vi "OE1022_Configure Input Filter.vi"(7 "OE1022_Configure Input Filter":T1 {"Input Notch Filter" items=["None"=0, "50Hz"=1, "100Hz"=3, "Both"=2]; "Input Coupling" items=["AC", "DC"]; "Input Shield Grounding" items=["Float", "Ground"]; "Input Source" items=["A", "A-B", "I-1M", "I-100M"]}, 8 "Error in (no error)":errorcluster caption="error out（no error）", 9 "Remote Mode":u16(ring) items=["USB"=0, "GPIB"=2], 11 "VISA resource name":refnum<visa-resource-name>) -> (0 "Error out":errorcluster caption="error out", 1 "Output String":string, 3 "VISA resource  out":refnum<visa-resource-name>)   [LabVIEW 2011]
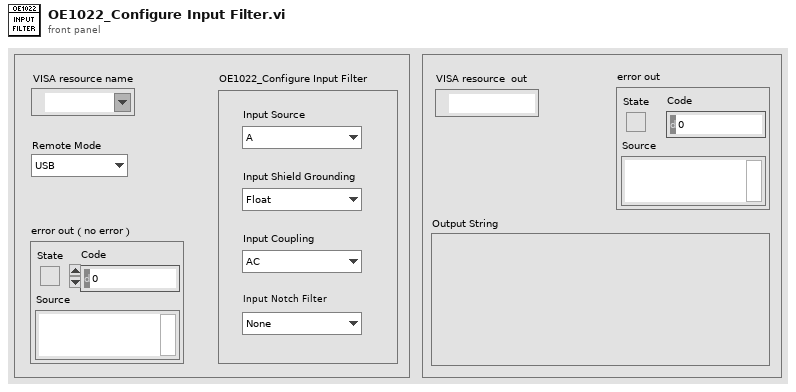
[diagram p1: front panel]
types:
  T1 = cluster{"Input Source":u16, "Input Shield Grounding ":u16, "Input Coupling ":u16, "Input Notch Filter ":u16}
  T2 = enum16{"ISRC", "IGND", "ICPL", "ILIN", "PHAS", "FMOD", "RSLP", "FREQ", "SWPT", "SLLM", "SULM", "SSLL", "SSLG", "STLM", "SWRM", "IRNG", "SENS", "RMOD", "OFLT", "OFSL", "SYNC", "DMOD", "HARM", "DARB", "SWVT", "SLVL", "SVLL", "SVUL", "SVSL", "SVSG", "SVTM", "SVRM", "RALL", "SNAP", "OUTP", "OAUX", "COUT", "CAUX", "COFP", "CEXP", "FPOP", "OEXP", "*IDN", "*RST", "OVLD", "INOV", "GNOV", "*PLL", "SSET", "RSET", "AGAN", "APHS", "ARSV", "ASCL", "EQCD", "EQCS", "SPED", "SRAT", "SLEN", "SSLE", "STRG", "SPRM", "STRD", "PAUS", "REST", "SPTS", "TRCA", "TEMP", "RSTU", "IHNZ", "DEQU", "SADD", "ARNG", "CSPE", "ISRCD", "IGNDD", "ICPLD", "ILIND", "PHASD", "FMODD", "RSLPD", "FREQD", "SWPTD", "SLLMD", "SULMD", "SSLLD", "SSLGD", "STLMD", "SWRMD", "SENSD", "RMODD", "OFLTD", "OFSLD", "SYNCD", "HARMD", "EQCDD", "EQCSD", "SNAPD", "OUTPD", "SWVTD", "SLVLD", "SVLLD", "SVULD", "SVSLD", "SVSGD", "SVTMD", "SVRMD", "SVDCD", "ARSVD", "AGAND", "APHSD", "ASCLD", "FPOPD", "CAUXD", "OEXPD", "SPEDD", "SRATD", "SLEND", "SSLED", "STRGD", "SPRMD", "STRDD", "PAUSD", "RESTD", "SPTSD", "TRCAD", "*IDND", "*RSTD", "INOVD", "GNOVD", "*PLLD", "SSETD", "RSETD"}
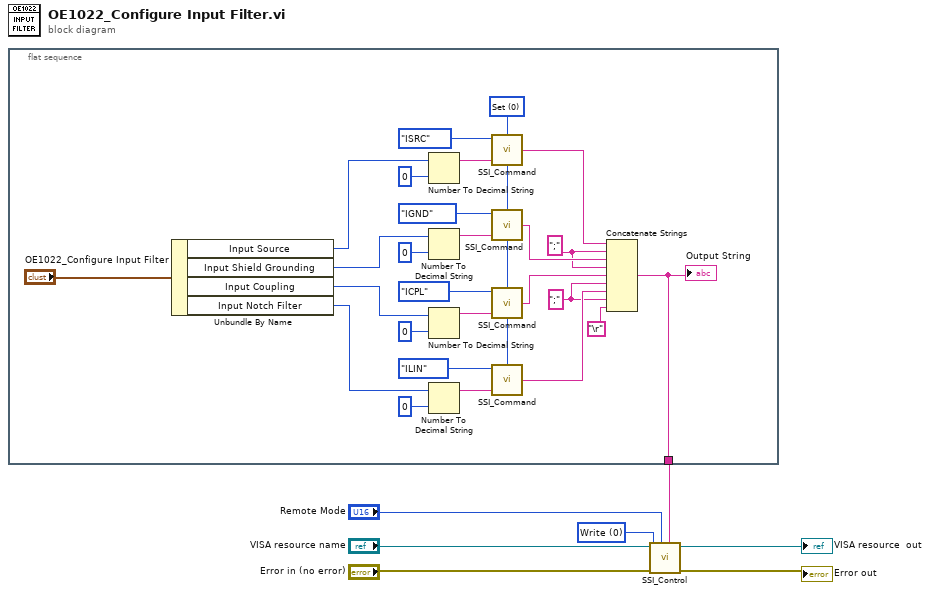
[diagram p0: block diagram]
diagram:
  w6 = u16 0 items=["Write", "Read"] ("Control")
  n1 = flat-sequence {
    tunnel: [w8] -> w1
    frame #0 {
      w10 = ";" ("字符串")
      w11 = ";" ("字符串")
      w28 = u16 0 items=["Set", "Query"] ("Opera")
      n2 = Unbundle By Name("OE1022_Configure Input Filter") -> ("Input Source"=w32:u16, "Input Shield Grounding"=w31:u16, "Input Coupling"=w30:u16, "Input Notch Filter"=w29:u16)
      n3 = Number To Decimal String(number=w32, width (-)=i16 0 ("精度(6)")) -> (decimal integer string=w26:string)
      n4 = Number To Decimal String(number=w31, width (-)=i16 0 ("精度(6)")) -> (decimal integer string=w23:string)
      n5 = Number To Decimal String(number=w30, width (-)=i16 0 ("精度(6)")) -> (decimal integer string=w18:string)
      n6 = Number To Decimal String(number=w29, width (-)=i16 0 ("精度(6)")) -> (decimal integer string=w15:string)
      n7 = call "SSI_Command.vi"("Opera"=w28, "Paramter"=w26, "Command Type"=T2."ISRC") -> ("Output string"=w21:string)  [unwired: 1 in]
      n8 = call "SSI_Command.vi"("Opera"=w28, "Paramter"=w23, "Command Type"=T2."IGND") -> ("Output string"=w20:string)  [unwired: 1 in]
      n9 = call "SSI_Command.vi"("Opera"=w28, "Paramter"=w18, "Command Type"=T2."ICPL") -> ("Output string"=w12:string)  [unwired: 1 in]
      n10 = call "SSI_Command.vi"("Opera"=w28, "Paramter"=w15, "Command Type"=T2."ILIN") -> ("Output string"=w13:string)  [unwired: 1 in]
      n11 = Concatenate Strings(w21, w11, w20, w11, w12, w10, w13, w10, "\r") -> (w8:string)
      "Output String" <- w8
    }
  }
  n12 = call "SSI_Control.vi"("Write Buffer"=w1, "Remote Mode"="Remote Mode", "Error in (no error)"="Error in (no error)", "Control"=w6, "VISA resource name"="VISA resource name") -> ("Error out"=→"Error out":errorcluster, "VISA resource  out"=→"VISA resource  out":refnum<visa-resource-name>)  [unwired: 3 in, 2 out]
